vi "Configure Burst.vi"(6 "Burst Count (5)":i32=5, 7 "Enable Burst (T: Enable)":bool=TRUE, 8 "error in (no error)":errorcluster, 9 "Burst Mode (0: Triggered)":u16(ring)=1 items=["Triggered", "Gated"], 10 "Channel (0: Channel 1)":T1 items=["Channel 1", "Channel 2"], 11 "VISA resource name":refnum<visa-resource-name>) -> (0 "error out":errorcluster, 3 "VISA resource name out":refnum<visa-resource-name>)   [LabVIEW 2023, in "Tektronix AFG 3000 Series.lvlib"]
doc: "Allows and configures burst modulation. Configures the function generator to output a waveform with specified number of cycles, called burst. The carrier waveform shape and parameters are set by Configure Standard Waveform."
uses:
  Tektronix AFG 3000 Series.lvlib
  controls.llb/Channel.ctl
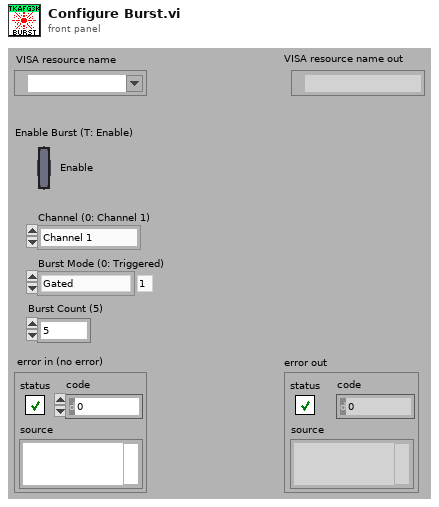
[diagram p1: front panel]
types:
  T1 = typedef "Channel.ctl" = u16
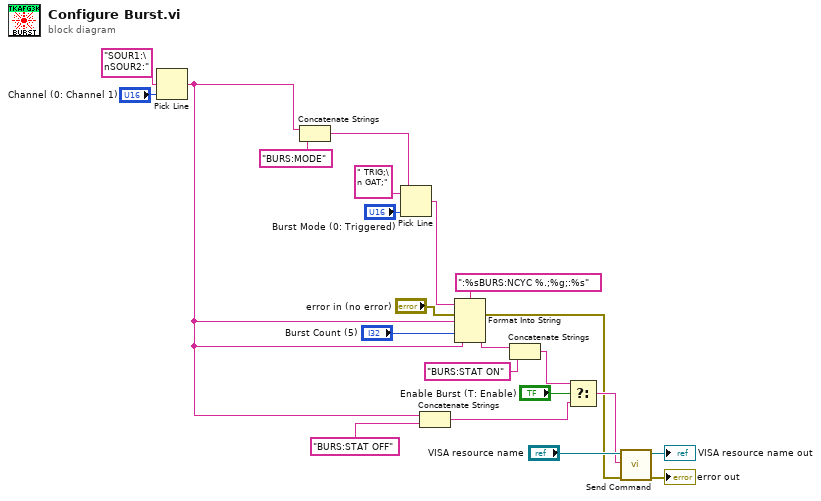
[diagram p0: block diagram]
diagram:
  n1 = Pick Line(multi-line string="SOUR1:\nSOUR2:" ("string (\"\")"), line index="Channel (0: Channel 1)") -> (output string=w7:string)  [unwired: 1 out]
  n2 = Concatenate Strings(w7, "BURS:MODE" ("format string")) -> (w10:string)
  n3 = Pick Line(string ("")=w10, multi-line string=" TRIG;\n GAT;" ("string (\"\")"), line index="Burst Mode (0: Triggered)") -> (output string=w12:string)
  n4 = Concatenate Strings(w7, "BURS:STAT OFF" ("string")) -> (w9:string)
  n5 = Format Into String(format string=":%sBURS:NCYC %.;%g;:%s", initial string=w12, error in="error in (no error)", w7, "Burst Count (5)", w7) -> (resulting string=w18:string, error out=w1:errorcluster)
  n6 = Concatenate Strings(w18, "BURS:STAT ON" ("string")) -> (w17:string)
  n7 = Select(t=w17, s="Enable Burst (T: Enable)", f=w9) -> (s? t:f=w2:string)
  n8 = call "Send Command.vi"("error in (no error)"=w1, "write buffer"=w2, "VISA resource name"="VISA resource name") -> ("error out"=→"error out":errorcluster, "VISA resource name out"=→"VISA resource name out":refnum<visa-resource-name>)  [unwired: 7 out]
